vi "tearDown.vi"(8 "error in (no error)":errorcluster, 11 "reference in":refnum<class "[Test Case] Create directory.lvclass">=refnum) -> (0 "error out":errorcluster, 3 "reference out":refnum<class "[Test Case] Create directory.lvclass">)   [LabVIEW 2016, in "Tests.lvlib" / "[Test Case] Create directory.lvclass"]
doc: "tearDown runs after the test method has completed. Use this method to clean up any operations or references that were opened by setUp or the test method. Unit tests should be independent of other unit tests so this VI should ensure that the next test can run in a 'clean' test environment."
uses:
  [Test Case] Create directory.lvclass
  classes/File Transfer Behavior/File Transfer Behavior.lvclass
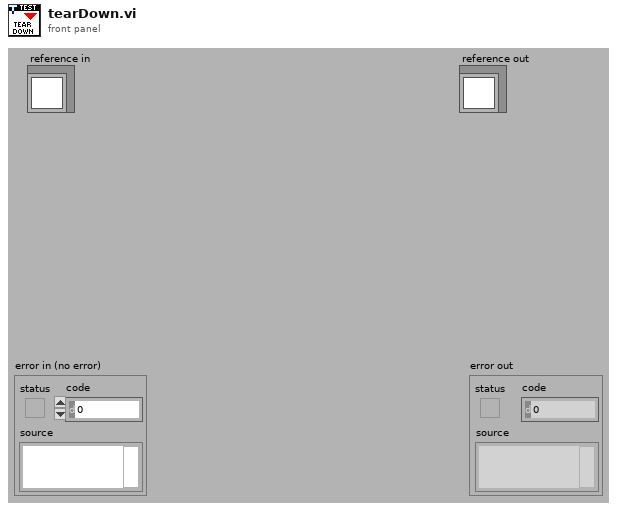
[diagram p1: front panel]
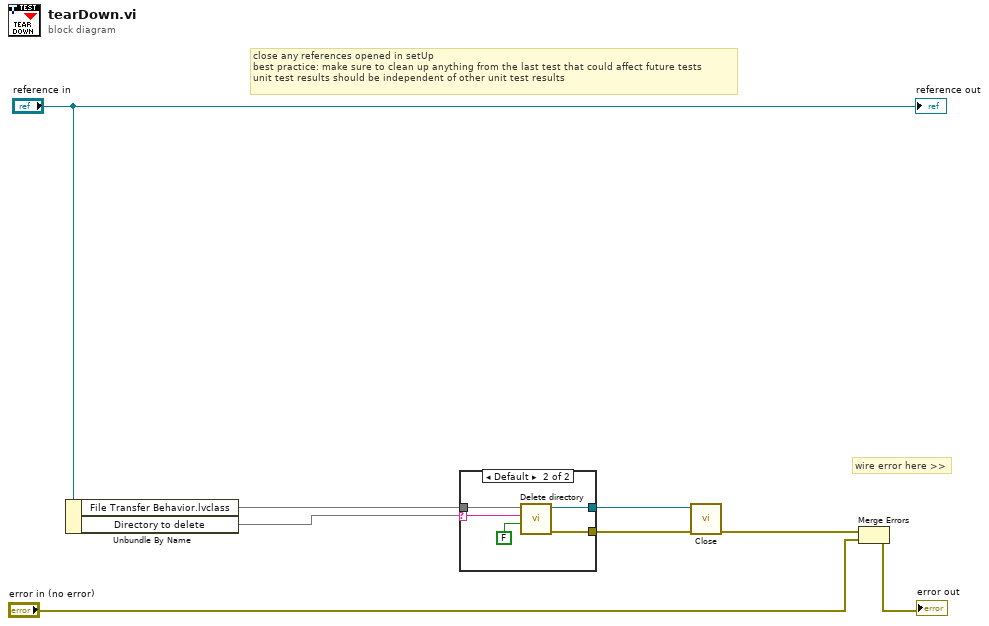
[diagram p0: block diagram]
diagram:
  # "wire error here >>"
  # "close any references opened in setUp\nbest practice: make sure to clean up anything from the last test that could affect future tests\nunit test results should be independent of other unit test results"
  n1 = Unbundle By Name("reference in") -> ("File Transfer Behavior.lvclass"=w2, "Directory to delete"=w1)
  n2 = case shown="Default" w1 {
    selector: w1 -> [_ w10]
    tunnel: [_ w14] -> w4
    tunnel: [w9 w13] -> w3
    tunnel: w2 -> [w9 w12]
    frame "" {
    }
    frame Default {
      n3 = call "Delete directory.vi"("Contents only? (true)"=FALSE, "Directory"=w10, "File Transfer Behavior in"=w12) -> ("error out"=w14:errorcluster, "File Transfer Behavior out"=w13:refnum<class "File Transfer Behavior.lvclass">)  [unwired: 7 in]
    }
  }
  n4 = call-dynamic "Close.vi"("error in (no error)"=w4, "File Transfer Behavior in"=w3) -> ("error out"=w5:errorcluster)  [unwired: 9 in]
  n5 = Merge Errors(w5, "error in (no error)") -> (→"error out":errorcluster)
  "reference out" <- "reference in"
